vi "PH_AxisGUI_BaseClass.Init FronPanel.vi"(0 "i ref in":refnum<vi>, 5 "error in":errorcluster) -> (14 "i ref out":refnum<vi>, 19 "error out":errorcluster)   [LabVIEW 2014, in "PH_AxisGUI_BaseClass.lvlib"]
doc: "This VI manipulates several GUI elements"
uses:
  PH_AxisGUI_BaseClass.lvlib
  PH_Common/PH_Common.lvlib
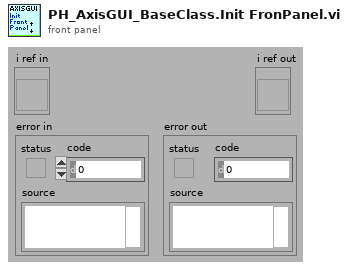
[diagram p1: front panel]
types:
  T1 = typedef "PH_AxisGUI_BaseClass.lvlib/PH_AxisGUI_BaseClass.i attribute.ctl" = cluster{"Axes":T2[]}
  T2 = typedef "PH_AxisGUI_BaseClass.lvlib/PH_AxisGUI_BaseClass.Axis Attributes.ctl" = cluster{"Axis GUI Refs":T3, "Address":T4, "Name":string, "Label \"Back\"":string, "Labell \"Forth\"":string, "Moving?":bool}
  T3 = typedef "PH_AxisGUI_BaseClass.lvlib/PH_AxisGUI_BaseClass.Axis GUI Refs.ctl" = cluster{"Back":refnum<vi>, "Forth":refnum<vi>, "Status":refnum<vi>, "Target":refnum<vi>, "Address":refnum<vi>, "Status Bar":refnum<vi>, "Settings":refnum<vi>, "Activity":refnum<vi>, "Clear Error":refnum<vi>}
  T4 = typedef "PH_Stepmotor_BaseClass.lvlib/PH_Stepmotor_BaseClass.Axis Address.ctl" = cluster{"Instance":string, "Motor Nr":i32}
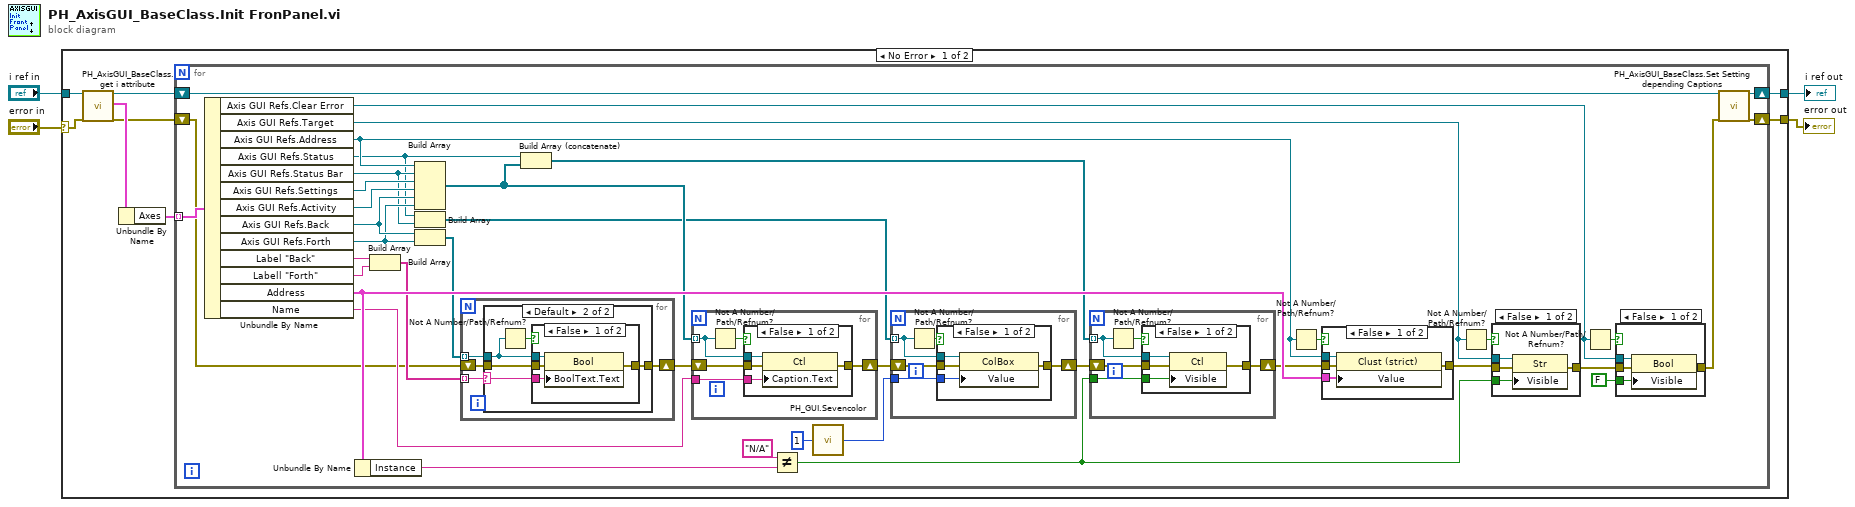
[diagram p0: block diagram]
diagram:
  n1 = case shown="No Error" "error in" {
    selector: "error in" -> [w10 w112]
    tunnel: "i ref in" -> [w12 w113]
    tunnel: [w11 w113] -> w3
    tunnel: [w5 w112] -> w1
    frame No Error {
      n2 = call "PH_AxisGUI_BaseClass.get i attribute.vi"("i ref in"=w12, "error in (no error)"=w10) -> ("i ref out"=w7:refnum<vi>, "i attribute"=w9:T1, "error out"=w6:errorcluster)  [unwired: 15 in]
      n3 = Unbundle By Name(w9) -> ("Axes"=w8:T2[])
      n4 = for {
        shift-right: [w41] -> w11
        shift-left: w7 -> [w42]
        shift-right: [w40] -> w5
        shift-left: w6 -> [w30]
        tunnel: w8 -> [w43] mode=indexing
        n5 = Unbundle By Name(w43) -> ("Axis GUI Refs.Clear Error"=w21:refnum<vi>, "Axis GUI Refs.Target"=w45:refnum<vi>, "Axis GUI Refs.Address"=w38:refnum<vi>, "Axis GUI Refs.Status"=w17:refnum<vi>, "Axis GUI Refs.Status Bar"=w18:refnum<vi>, "Axis GUI Refs.Settings"=w51:refnum<vi>, "Axis GUI Refs.Activity"=w48:refnum<vi>, "Axis GUI Refs.Back"=w37:refnum<vi>, "Axis GUI Refs.Forth"=w36:refnum<vi>, "Label \"Back\""=w34:string, "Labell \"Forth\""=w35:string, "Address"=w39:T4, "Name"=w31:string)
        n6 = Unbundle By Name(w39) -> ("Instance"=w44:string)
        n7 = Build Array(w34, w35) -> (w32:string[])
        n8 = Build Array(w38, w18, w51, w48, w37, w36) -> (w27:refnum<vi>[])
        n9 = Build Array(w17, w18) -> (w16:refnum<vi>[])
        n10 = Build Array(w37, w36) -> (w33:refnum<vi>[])
        n11 = for {
          shift-right: [w80] -> w29
          shift-left: w30 -> [w79]
          tunnel: w33 -> [w78] mode=indexing
          tunnel: w32 -> [w77] mode=indexing
          n12 = case shown="Default" w77 {
            selector: w77 -> [_ w82]
            tunnel: [w81 w86] -> w80
            tunnel: w79 -> [w81 w85]
            tunnel: w78 -> [_ w84]
            frame "", "N/A" {
            }
            frame Default {
              n13 = Not A Number/Path/Refnum?(number/path/refnum=w84) -> (NaN/Path/Refnum?=w83:bool)
              n14 = case shown="False" w83 {
                tunnel: [w90 w91] -> w86
                tunnel: w85 -> [w89 w91]
                tunnel: w84 -> [w88 _]
                tunnel: w82 -> [w87 _]
                frame False {
                  n15 = property class="Bool"(reference=w88, error in=w89, "BoolText.Text"=w87) -> (error out=w90:errorcluster)  [unwired: 1 out]
                }
                frame True {
                }
              }
            }
          }
        }
        n16 = Build Array (concatenate)(w17, w27) -> (w26:refnum<vi>[])
        n17 = for {
          tunnel: w27 -> [w93] mode=indexing
          shift-right: [w92] -> w20
          shift-left: w29 -> [w96]
          tunnel: w31 -> [w95]
          n18 = Not A Number/Path/Refnum?(number/path/refnum=w93) -> (NaN/Path/Refnum?=w94:bool)
          n19 = case shown="False" w94 {
            tunnel: w93 -> [w100 _]
            tunnel: w96 -> [w99 w101]
            tunnel: w95 -> [w98 _]
            tunnel: [w97 w101] -> w92
            frame False {
              n20 = property class="Ctl"(reference=w100, error in=w99, "Caption.Text"=w98) -> (error out=w97:errorcluster)  [unwired: 1 out]
            }
            frame True {
            }
          }
        }
        n21 = Not Equal?(x="N/A", y=w44) -> (x != y?=w22:bool)
        n22 = call "PH_GUI.Sevencolor.vi"("State"=1) -> ("Color Box"=w14:u32)
        n23 = for {
          tunnel: w16 -> [w53] mode=indexing
          shift-right: [w52] -> w19
          shift-left: w20 -> [w56]
          tunnel: w14 -> [w55]
          n24 = Not A Number/Path/Refnum?(number/path/refnum=w53) -> (NaN/Path/Refnum?=w54:bool)
          n25 = case shown="False" w54 {
            tunnel: w53 -> [w60 _]
            tunnel: w56 -> [w59 w61]
            tunnel: w55 -> [w57 _]
            tunnel: [w58 w61] -> w52
            frame False {
              n26 = property class="ColBox"(reference=w60, error in=w59, "Value"=w57) -> (error out=w58:errorcluster)  [unwired: 1 out]
            }
            frame True {
            }
          }
        }
        n27 = for {
          tunnel: w26 -> [w68] mode=indexing
          shift-right: [w67] -> w28
          shift-left: w19 -> [w71]
          tunnel: w22 -> [w70]
          n28 = Not A Number/Path/Refnum?(number/path/refnum=w68) -> (NaN/Path/Refnum?=w69:bool)
          n29 = case shown="False" w69 {
            tunnel: w68 -> [w75 _]
            tunnel: w71 -> [w74 w76]
            tunnel: w70 -> [w73 _]
            tunnel: [w72 w76] -> w67
            frame False {
              n30 = property class="Ctl"(reference=w75, error in=w74, "Visible"=w73) -> (error out=w72:errorcluster)  [unwired: 1 out]
            }
            frame True {
            }
          }
        }
        n31 = Not A Number/Path/Refnum?(number/path/refnum=w38) -> (NaN/Path/Refnum?=w49:bool)
        n32 = case "Config Axis Controls" shown="False" w49 {
          tunnel: w39 -> [w109 _]
          tunnel: [w110 w111] -> w47
          tunnel: w28 -> [w108 w111]
          tunnel: w38 -> [w107 _]
          frame False {
            n33 = property class="Clust (strict)"(reference=w107, error in=w108, "Value"=w109) -> (error out=w110:errorcluster)  [unwired: 1 out]
          }
          frame True {
          }
        }
        n34 = Not A Number/Path/Refnum?(number/path/refnum=w45) -> (NaN/Path/Refnum?=w46:bool)
        n35 = case "Config Axis Controls" shown="False" w46 {
          tunnel: w47 -> [w105 w106]
          tunnel: w45 -> [w104 _]
          tunnel: [w103 w106] -> w24
          tunnel: w22 -> [w102 _]
          frame False {
            n36 = property class="Str"(reference=w104, error in=w105, "Visible"=w102) -> (error out=w103:errorcluster)  [unwired: 1 out]
          }
          frame True {
          }
        }
        n37 = Not A Number/Path/Refnum?(number/path/refnum=w21) -> (NaN/Path/Refnum?=w25:bool)
        n38 = case "Config Axis Controls" shown="False" w25 {
          tunnel: w24 -> [w65 w66]
          tunnel: w21 -> [w64 _]
          tunnel: [w63 w66] -> w23
          tunnel: FALSE -> [w62 _]
          frame False {
            n39 = property class="Bool"(reference=w64, error in=w65, "Visible"=w62) -> (error out=w63:errorcluster)  [unwired: 1 out]
          }
          frame True {
          }
        }
        n40 = call "PH_AxisGUI_BaseClass.Set Setting depending Captions.vi"("i ref out"=w42, "error in"=w23) -> ("i ref out"=w41:refnum<vi>, "error out"=w40:errorcluster)  [unwired: 16 in]
      }
    }
    frame Error {
    }
  }
  "error out" <- w1
  "i ref out" <- w3
